vi "Preset START WAIT Time query.vi"(8 "error in (no error)":errorcluster, 11 "VISA resource in":refnum<visa-resource-name>) -> (0 "error out":errorcluster, 2 "Time":string, 3 "VISA resource out":refnum<visa-resource-name>)   [LabVIEW 2025, in "Chroma 19572.lvlib"]
doc: "This VI writes to the instrument the AUTO RANGE state."
uses:
  <instrlib>/Chroma 19572/Chroma 19572.lvlib
panel:
  # "0 = OFF\n0,1 to 99,9 sec"
  # "PreSet START WAIT time befor GB test"
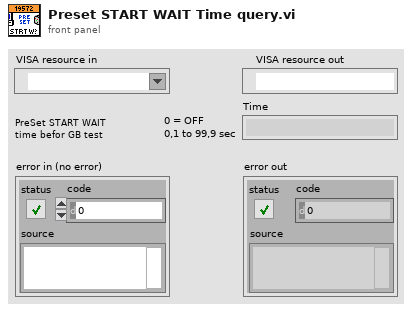
[diagram p1: front panel]
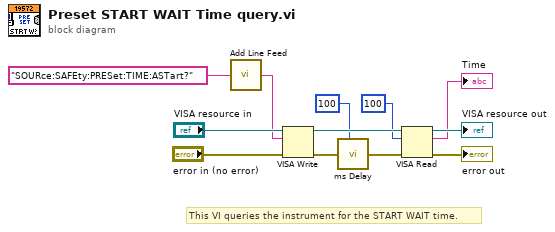
[diagram p0: block diagram]
diagram:
  # "This VI queries the instrument for the START WAIT time."
  n1 = call <instrlib>:"Add Line Feed.vi"("Command string"="SOURce:SAFEty:PRESet:TIME:ASTart?") -> ("Concatenated string"=w8:string)  [unwired: 4 in]
  n2 = VISA Write(VISA resource name="VISA resource in", write buffer=w8, error in (no error)="error in (no error)") -> (VISA resource name out=w12:refnum<visa-resource-name>, error out=w3:errorcluster)  [unwired: 1 out]
  n3 = call <instrlib>:"ms Delay.vi"("miliseconds to wait"=u32 100, "error in (no error)"=w3) -> ("error out"=w7:errorcluster)  [unwired: 6 in, 1 out]
  n4 = VISA Read(VISA resource name=w12, byte count=u32 100, error in (no error)=w7) -> (VISA resource name out=→"VISA resource out":refnum<visa-resource-name>, read buffer=→"Time":string, error out=→"error out":errorcluster)  [unwired: 1 out]
